vi "status of worker3.vi"() -> ()   [LabVIEW 2020]
panel:
  out "worker3_busy/ready":bool
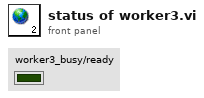
[diagram p1: front panel]
diagram:
